vi "Switch Hydrogen Sensor Mode.vi"(0 "Session Handle":T1, 5 "Modbus?":bool, 11 "error in (no error)":errorcluster) -> (4 "Session Handle Out":T1, 15 "error out":errorcluster)   [LabVIEW 2015, in "Peltier.lvclass"]
uses:
  Peltier.lvclass
  Typedefs/Session Handle.ctl
  Gas/Gas.lvclass
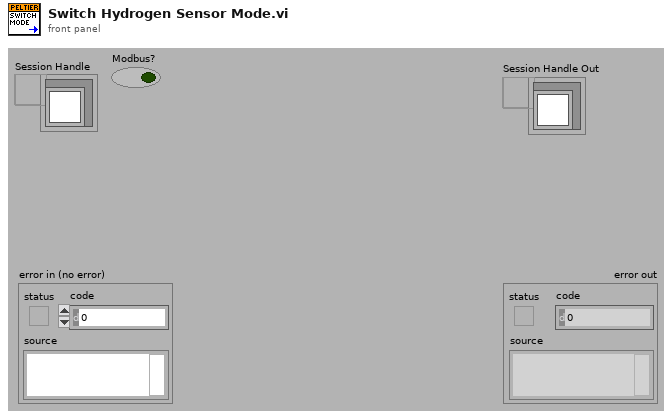
[diagram p1: front panel]
types:
  T1 = typedef "Peltier.lvclass/Session Handle.ctl" = refnum<data-value>
  T2 = typedef "XNET Frame CAN.ctl" = cluster{"timestamp":timestamp, "payload":u8[], "identifier":u32, "type":T3, "extended?":bool, "echo?":bool}
  T3 = typedef "XNET Frame Type CAN.ctl" = u8
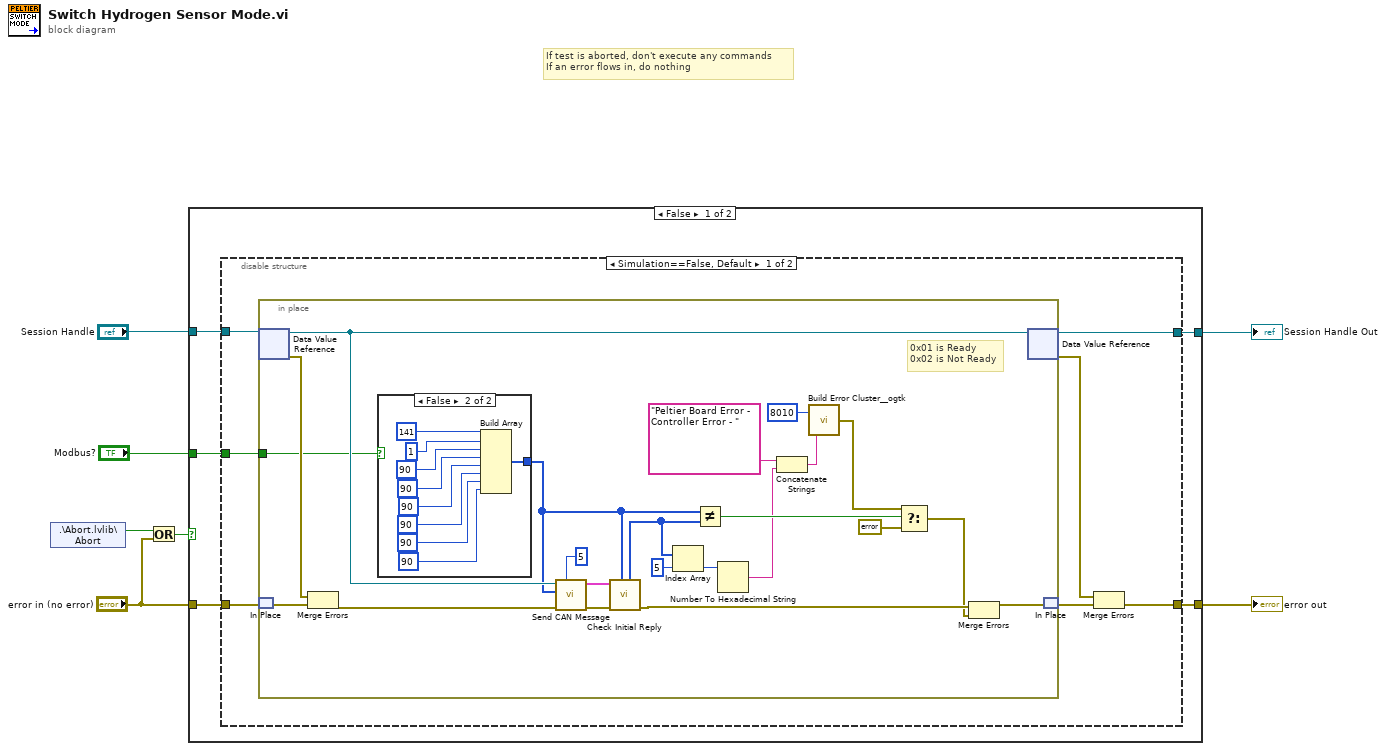
[diagram p0: block diagram]
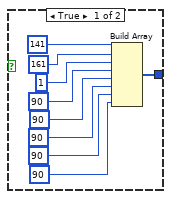
[diagram p2: hidden frame]
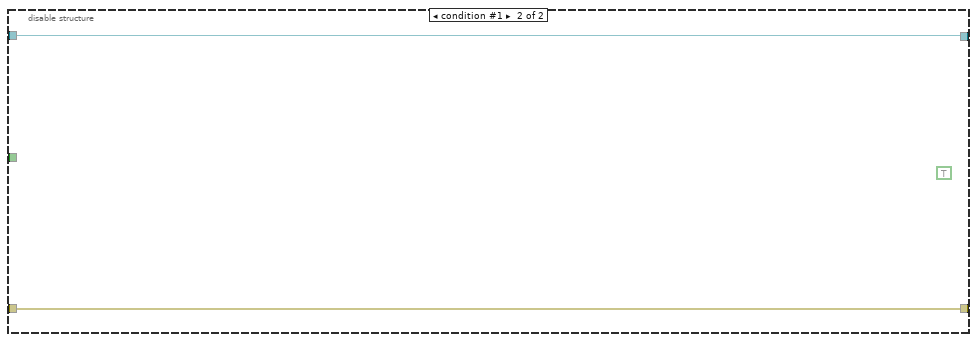
[diagram p3: hidden frame]
diagram:
  # "If test is aborted, don't execute any commands\nIf an error flows in, do nothing"
  n1 = shared-variable ".\\Abort.lvlib\\Abort"() -> (w6:bool)  [unwired: 1 in, 1 out]
  n2 = Or(x=w6, y="error in (no error)") -> (x .or. y?=w4:bool)
  n3 = case shown="False" w4 {
    tunnel: [w12 w63] -> w2
    tunnel: [w11 w62] -> w7
    tunnel: "Session Handle" -> [w10 w63]
    tunnel: "error in (no error)" -> [w9 w62]
    tunnel: "Modbus?" -> [w8 _]
    frame False {
      n4 = disable-structure shown="Simulation==False, Default" {
        disable-tunnel: [w19 w61] -> w12
        disable-tunnel: [w16 w60] -> w11
        disable-tunnel: w10 -> [w15 w61]
        disable-tunnel: w9 -> [w14 w60]
        disable-tunnel: w8 -> [w13 _]
        frame condition #0 (active) {
          n5 = in-place {
            in-place-border: w13 -> [w31]
            # "0x01 is Ready\n0x02 is Not Ready"
            n6 = in-place-dvr #1(w15) -> (w32:refnum<class "Peltier.lvclass">, w40:errorcluster)
            n7 = in-place-match #2(w14) -> (w39:errorcluster)
            n8 = Merge Errors(w40, w39) -> (w38:errorcluster)
            n9 = case shown="False" w31 {
              tunnel: [w42 w51] -> w30
              frame True {
                n10 = Build Array(u8 141 ("new element/subarray"), u8 161 ("new element/subarray"), u8 1 ("new element/subarray"), u8 90 ("new element/subarray"), u8 90 ("new element/subarray"), u8 90 ("new element/subarray"), u8 90 ("new element/subarray"), u8 90 ("new element/subarray")) -> (w42:u8[])
              }
              frame False {
                n11 = Build Array(u8 141 ("new element/subarray"), u8 1 ("new element/subarray"), u8 90 ("new element/subarray"), u8 90 ("new element/subarray"), u8 90 ("new element/subarray"), u8 90 ("new element/subarray"), u8 90 ("new element/subarray"), u8 90 ("new element/subarray")) -> (w51:u8[])
              }
            }
            n12 = call "Send CAN Message.vi"("Number of Retries"=5, "error in (no error)"=w38, "payload"=w30, "Peltier In"=w32) -> ("error out"=w22:errorcluster, "Reply"=w36:T2[])  [unwired: 5 in, 1 out]
            n13 = call "Check Initial Reply.vi"("Write Message"=w30, "error in (no error)"=w22, "Reply"=w36) -> ("error out"=w21:errorcluster, "Whole Payload"=w28:u8[])  [unwired: 5 in, 2 out]
            n14 = Index Array(array=w28, index=5) -> (element=w26:u8)
            n15 = Not Equal?(x=w30, y=w28) -> (x != y?=w29:bool)
            n16 = Number To Hexadecimal String(2:w26) -> (0:w24:string)  [unwired: 1 in]
            n17 = Concatenate Strings("Peltier Board Error - Controller Error - " ("string"), w24) -> (w23:string)
            n18 = call <userlib>:"Build Error Cluster__ogtk.vi"("String to Prepend to source (\"\")"=w23, "code"=8010) -> ("error out"=w34:errorcluster)
            n19 = Select(t=w34, s=w29, f=errorcluster {"status"=FALSE, "code"=0, "source"=""}) -> (s? t:f=w20:errorcluster)
            n20 = Merge Errors(w21, w20) -> (w41:errorcluster)
            n21 = in-place-dvr #1(w32) -> (w19:T1, w17:errorcluster)
            n22 = in-place-match #2(w41) -> (w18:errorcluster)
          }
          n23 = Merge Errors(w17, w18) -> (w16:errorcluster)
        }
        frame condition #1 {
          (unwired) TRUE
        }
      }
    }
    frame True {
    }
  }
  "error out" <- w7
  "Session Handle Out" <- w2
